vi "ClearAvailableRecords.vi"(8 "error in (no error)":errorcluster, 11 "Scope5785_six_channel":refnum<class "Scope5782_six_channel.lvclass">) -> (0 "error out":errorcluster, 3 "Scope5785_six_channel out":refnum<class "Scope5782_six_channel.lvclass">)   [LabVIEW 2018, in "Scope5782_six_channel.lvclass"]
uses:
  Scope5782_six_channel.lvclass
  Scope5782_six_channel.lvclass/Scope5782_six_channel.ctl
  FpgaRef/FpgaRef5761/FpgaRef5761.lvclass
  FpgaRef/FpgaRef5782/FpgaRef5782.lvclass
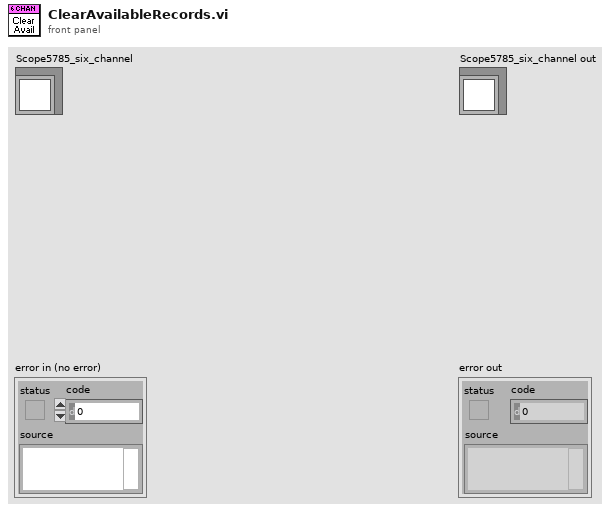
[diagram p1: front panel]
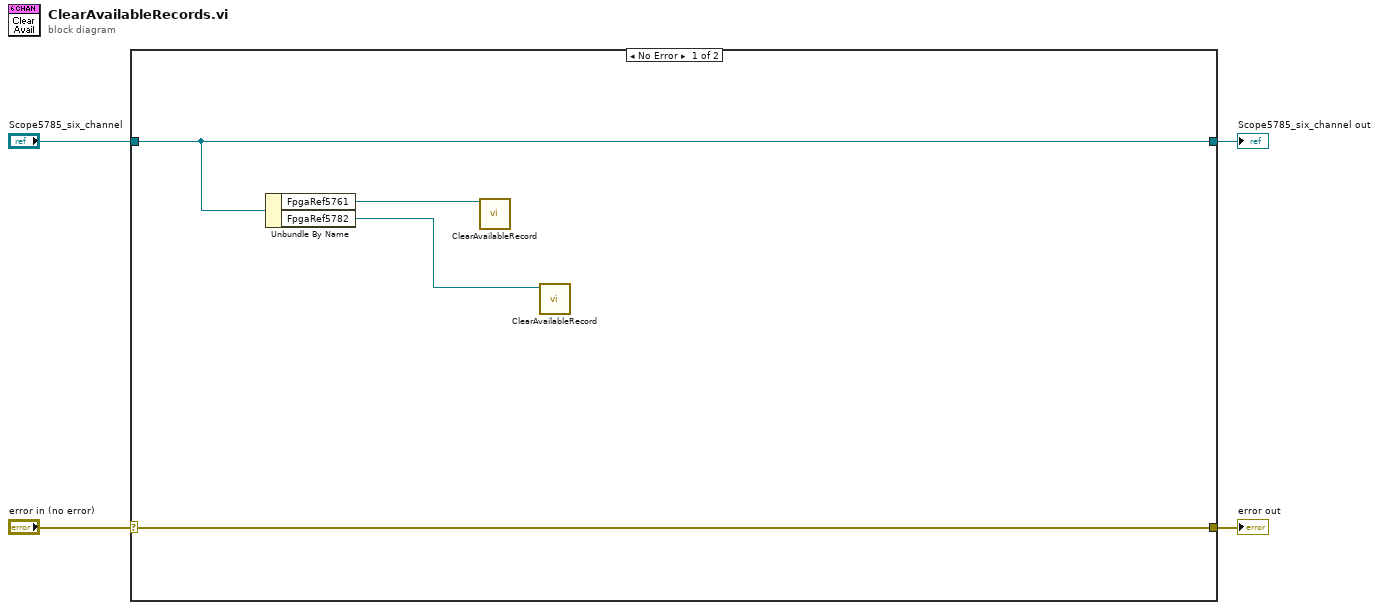
[diagram p0: block diagram]
diagram:
  n1 = case shown="No Error" "error in (no error)" {
    selector: "error in (no error)" -> [w8 w10]
    tunnel: [w8 w10] -> w3
    tunnel: [w7 w9] -> w1
    tunnel: "Scope5785_six_channel" -> [w7 w9]
    frame No Error {
      n2 = Unbundle By Name(w7) -> ("FpgaRef5761"=w6:refnum<class "FpgaRef5761.lvclass">, "FpgaRef5782"=w5:refnum<class "FpgaRef5782.lvclass">)
      n3 = call "ClearAvailableRecord.vi"("FpgaRef5761 in"=w6) -> ()  [unwired: 9 in, 2 out]
      n4 = call "ClearAvailableRecord.vi"("FpgaRef5782 In"=w5) -> ()  [unwired: 9 in, 2 out]
    }
    frame Error {
    }
  }
  "error out" <- w3
  "Scope5785_six_channel out" <- w1
